vi "levelTank.vi"(10 "Alarm Level":dbl(slide) scale=0.0..10.0, 11 "Select level":dbl(slide) scale=0.0..10.0) -> (1 "Message":string, 2 "Alarm Activated":bool, 3 "Fuel Level":dbl(slide) scale=0.0..10.0)   [LabVIEW 2014]
doc: "This VI allow you to explore indicators and controls in a Labview program."
panel:
  in  "stop":bool
  # "Vi for fuel level monitoring"
  # "1. Select the value for alarm in the control called \"Alarm Level.\n2. Uses the control \"Select level\" and test the system changind the level, for greater values of alarm level,  the system must show an alarm message and also turn ON the Led \"Alarm Activated.\nver como se activa el indicador luminoso.\n3. Test the program and after click in the stop button."
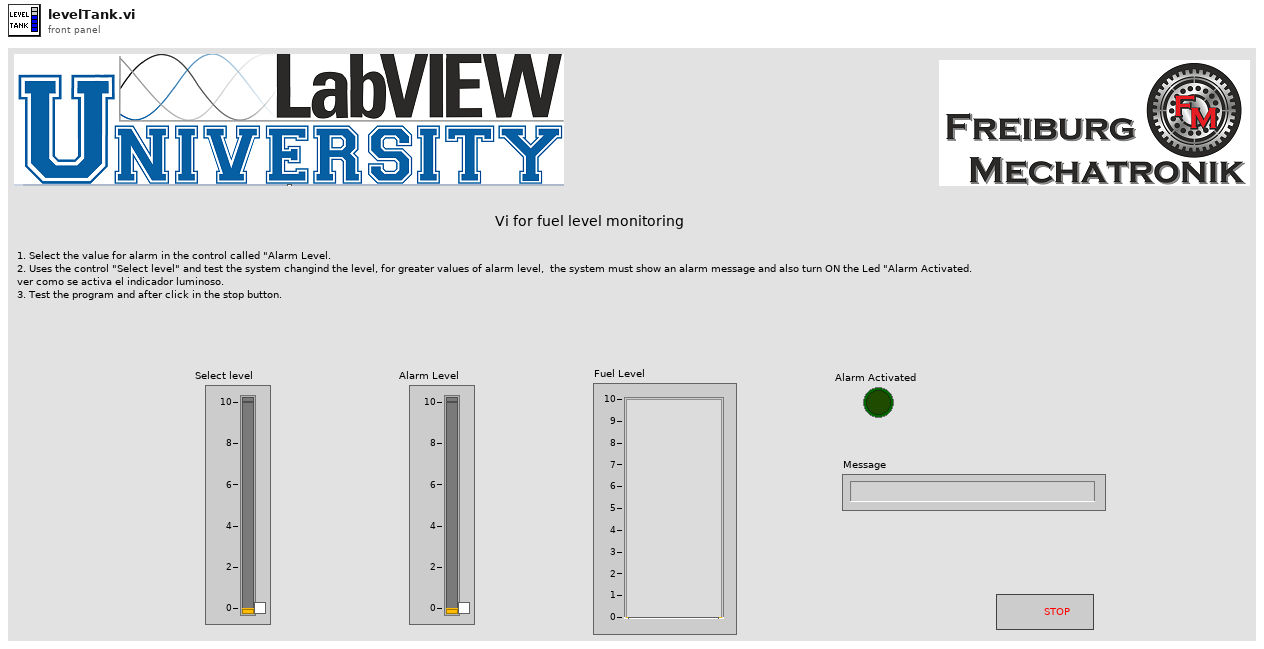
[diagram p1: front panel]
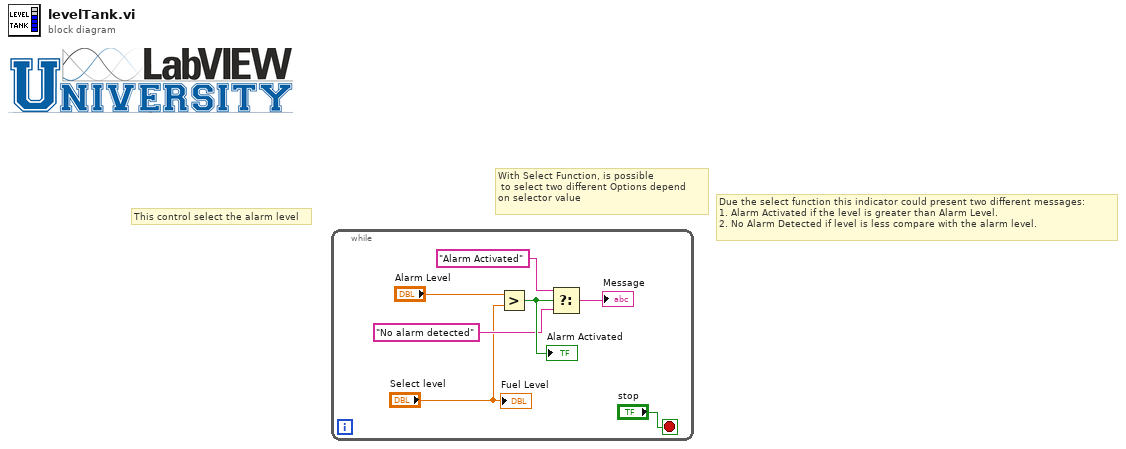
[diagram p0: block diagram]
diagram:
  # "With Select Function, is possible\n to select two different Options depend \non selector value"
  # "This control select the alarm level"
  # "Due the select function this indicator could present two different messages:\n1. Alarm Activated if the level is greater than Alarm Level.\n2. No Alarm Detected if level is less compare with the alarm level."
  n1 = while {
    stop <- "stop" stop-if-true
    n2 = Greater?(x="Alarm Level", y="Select level") -> (0:w5:bool)
    "Alarm Activated" <- w5
    n3 = Select(t="Alarm Activated", s=w5, f="No alarm detected") -> (s? t:f=→"Message":string)
    "Fuel Level" <- "Select level"
  }
